vi "KE622x -- Set Arm Output Mode.vi"(0 "Resource In":refnum<visa-resource-name>, 1 "Check For SCPI Errors? (T)":bool=TRUE, 7 "Arm Output Mode":T1, 11 "error in (no error)":errorcluster) -> (4 "Resource Out (dupl)":refnum<visa-resource-name>, 15 "error out":errorcluster)   [LabVIEW 2018, in "Keithley 622x.lvlib"]
uses:
  Keithley 622x.lvlib
  Typedefs/KE622x -- Arm Output Mode.ctl
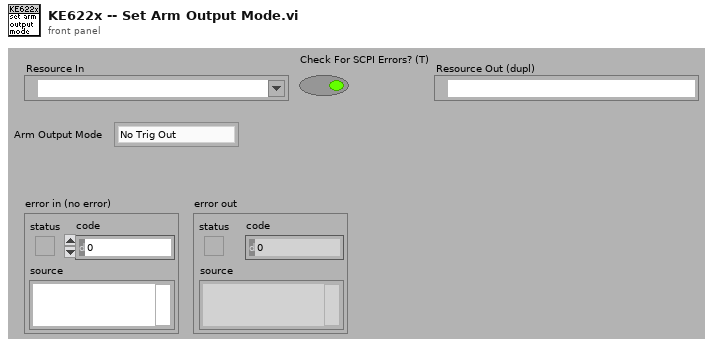
[diagram p1: front panel]
types:
  T1 = typedef "Keithley 622x.lvlib/KE622x -- Arm Output Mode.ctl" = enum16{"No Trig Out", "Trig Out On Enter Arm", "Trig Out On Exit Arm"}
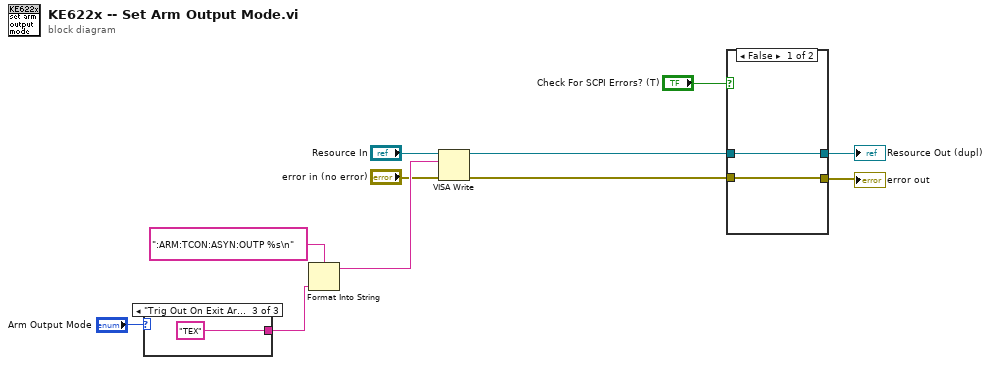
[diagram p0: block diagram]
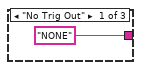
[diagram p2: hidden frame]
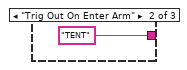
[diagram p3: hidden frame]
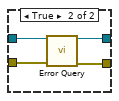
[diagram p4: hidden frame]
diagram:
  n1 = case shown="\"Trig Out On Exit Arm\"" "Arm Output Mode" {
    tunnel: ["NONE" "TENT" "TEX"] -> w3
    frame "No Trig Out" {
    }
    frame "Trig Out On Enter Arm" {
    }
    frame "Trig Out On Exit Arm" {
    }
  }
  n2 = Format Into String(format string=":ARM:TCON:ASYN:OUTP %s\n", w3) -> (resulting string=w9:string)  [unwired: 2 in, 1 out]
  n3 = VISA Write(VISA resource name="Resource In", write buffer=w9, error in (no error)="error in (no error)") -> (VISA resource name out=w6:refnum<visa-resource-name>, error out=w5:errorcluster)  [unwired: 1 out]
  n4 = case shown="False" "Check For SCPI Errors? (T)" {
    tunnel: w6 -> [w16 w20]
    tunnel: w5 -> [w15 w19]
    tunnel: [w15 w18] -> w1
    tunnel: [w16 w17] -> w2
    frame False {
    }
    frame True {
      n5 = call "Error Query.vi"("VISA Resource In"=w20, "error in (no error)"=w19) -> ("VISA Resource Out (dupl)"=w17:refnum<visa-resource-name>, "error out"=w18:errorcluster)  [unwired: 10 in, 2 out]
    }
  }
  "Resource Out (dupl)" <- w2
  "error out" <- w1
